vi "RMS_ACV.vi"(9 "# of samples":dbl, 10 "Vave":dbl, 11 "Data IN":dbl[](array[numeric])) -> (3 "VRMS":dbl)   [LabVIEW 2012]
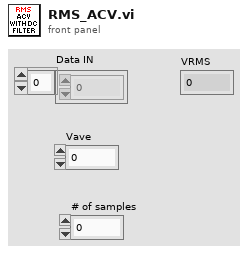
[diagram p1: front panel]
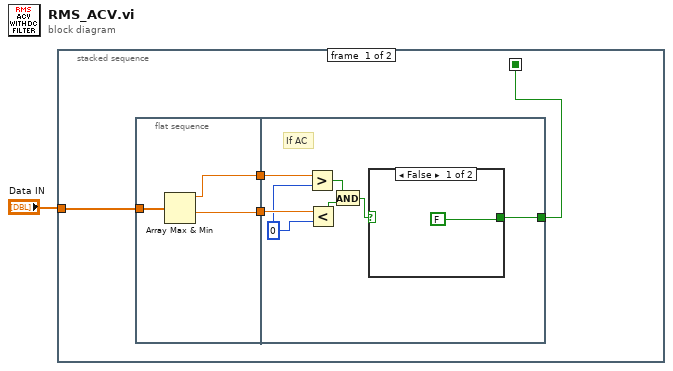
[diagram p0: block diagram]
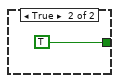
[diagram p2: hidden frame]
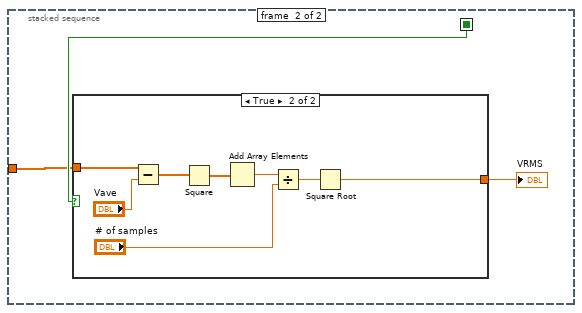
[diagram p3: hidden frame]
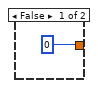
[diagram p4: hidden frame]
diagram:
  n1 = stacked-sequence {
    seq-local: [w2 _] -> [_ w19]
    tunnel: "Data IN" -> [w3 w18]
    frame #0 {
      n2 = flat-sequence {
        tunnel: [w8] -> w5
        tunnel: [w7] -> w4
        tunnel: w3 -> [w6]
        tunnel: [w15] -> w2
        tunnel: w5 -> [w14]
        tunnel: w4 -> [w12]
        frame #0 {
          n3 = Array Max & Min(array=w6) -> (max value=w7:dbl, min value=w8:dbl)  [unwired: 2 out]
        }
        frame #1 {
          w13 = 0
          # "If AC"
          n4 = Greater?(x=w12, y=w13) -> (0:w10:bool)
          n5 = Less?(x=w14, y=w13) -> (x < y?=w9:bool)
          n6 = And(x=w10, y=w9) -> (x .and. y?=w11:bool)
          n7 = case shown="False" w11 {
            tunnel: [FALSE TRUE] -> w15
            frame False {
            }
            frame True {
            }
          }
        }
      }
    }
    frame #1 {
      n8 = case shown="True" w19 {
        tunnel: w18 -> [_ w25]
        tunnel: [0 w22] -> w20
        frame False {
        }
        frame True {
          n9 = Subtract(x=w25, y="Vave") -> (x-y=w26:dbl[])
          n10 = Square(x=w26) -> (x^2=w27:dbl[])
          n11 = Add Array Elements(numeric array=w27) -> (sum=w28:dbl)
          n12 = Divide(x=w28, y="# of samples") -> (x/y=w29:dbl)
          n13 = Square Root(x=w29) -> (sqrt(x)=w22:dbl)
        }
      }
      "VRMS" <- w20
    }
  }
